vi "Generate PWM Waveform.vi"(4 "PWM Ratio Min":dbl format="%.3g", 5 "PWM Sample Rate":dbl[unit]=1000.0, 6 "PWM Ratio Max":dbl format="%.3g", 7 "PWM Length":dbl[unit]=1.0 format="%.3g", 8 "error in (no error)":errorcluster, 9 "PWM Delay":dbl format="%.3g", 10 "PWM Ratio":dbl format="%.3g", 11 "Timestamp":timestamp) -> (0 "error out":errorcluster, 3 "PWM Waveform":waveform(dbl))   [LabVIEW 2020, in "BNT_ULx.lvlib" / "BNT_ULx-MCSV-DOPWM.lvclass"]
doc: "Generate waveform from PWM Ratio and Delay."
uses:
  BNT_ULx-MCSV-DOPWM.lvclass
  BNT_ULx-MCSV-DOPWM.lvclass/BNT_ULx-MCSV-DOPWM.ctl
  <vilib>/Analysis/NI_AALBase.lvlib
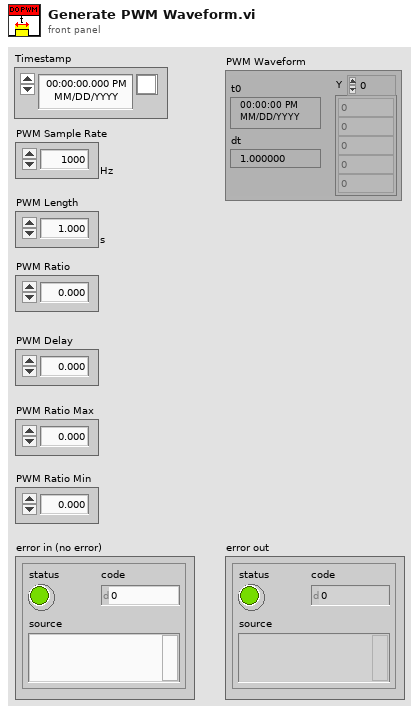
[diagram p1: front panel]
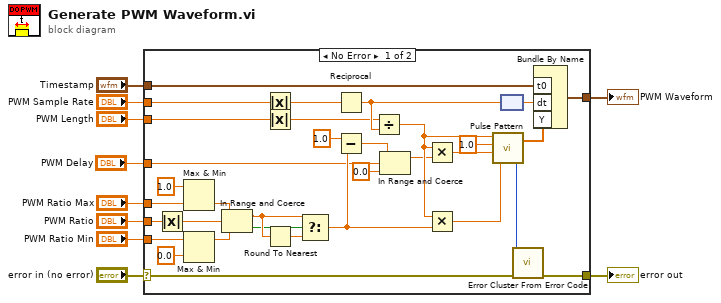
[diagram p0: block diagram]
diagram:
  n1 = case shown="No Error" "error in (no error)" {
    selector: "error in (no error)" -> [w35 w44]
    tunnel: "PWM Delay" -> [w39 _]
    tunnel: "PWM Ratio" -> [w32 _]
    tunnel: "PWM Length" -> [w29 _]
    tunnel: "PWM Sample Rate" -> [w28 _]
    tunnel: [w26 w44] -> w5
    tunnel: [w25 _] -> w4
    tunnel: "Timestamp" -> [w24 _]
    tunnel: "PWM Ratio Max" -> [w19 _]
    tunnel: "PWM Ratio Min" -> [w16 _]
    frame No Error {
      n2 = Absolute Value(x=w32) -> (abs(x)=w11:dbl)
      n3 = Max & Min(x=1.0, y=w19) -> (min(x,y)=w17:dbl)  [unwired: 1 out]
      n4 = Max & Min(x=w16, y=0.0) -> (max(x,y)=w15:dbl)  [unwired: 1 out]
      n5 = In Range and Coerce(upper limit=w17, x=w11, lower limit=w15) -> (coerced(x)=w34:dbl, In Range?=w33:bool)
      n6 = Absolute Value(x=w28) -> (abs(x)=w12:dbl[unit])
      n7 = Absolute Value(x=w29) -> (abs(x)=w13:dbl[unit])
      n8 = Round To Nearest(number=w34) -> (nearest integer value=w31:dbl)
      n9 = Select(t=w34, s=w33, f=w31) -> (s? t:f=w41:dbl)
      n10 = Reciprocal(x=w12) -> (1/x=w30:dbl[unit])
      n11 = Subtract(x=1.0, y=w41) -> (x-y=w36:dbl)
      n12 = Divide(x=w13, y=w30) -> (x/y=w43:dbl)
      n13 = In Range and Coerce(upper limit=w36, x=w39, lower limit=0.0) -> (coerced(x)=w40:dbl)  [unwired: 1 out]
      n14 = Multiply(x=w43, y=w40) -> (x*y=w42:dbl)
      n15 = Multiply(x=w43, y=w41) -> (x*y=w21:dbl)
      n16 = call <vilib>:"Pulse Pattern.vi"("width"=w21, "delay"=w42, "amplitude"=1.0, "samples"=w43) -> ("error"=w22:i32, "Pulse Pattern"=w23:dbl[])
      n17 = node(w30) -> (w27:dbl)
      n18 = call <vilib>:"Error Cluster From Error Code.vi"("error in (no error)"=w35, "error code (0)"=w22) -> ("error out"=w26:errorcluster)  [unwired: 7 in]
      n19 = Bundle By Name("t0"=w24, "dt"=w27, "Y"=w23) -> (w25:waveform(dbl))  [unwired: 1 in]
    }
    frame Error {
    }
  }
  "error out" <- w5
  "PWM Waveform" <- w4
